vi "oa_Buffer and Compute Orbit Plot Data.vi"(5 "reset? (F)":bool, 6 "trigger pulse direction":u16(ring)=1 items=["positive going", "negative going"], 7 "tach duty":i32=1, 8 "actual samples/rev":dbl format="%.2f", 9 "revolutions":dbl format="%.2f", 10 "start":dbl format="%.2f", 11 "order waveform":dbl[][](array[numeric]) format="%.2f") -> (3 "orbit data":cluster{dbl[], dbl[]}[](array[cluster]) {"?" format="%.2f"; "?" format="%.2f"})   [LabVIEW 2017]
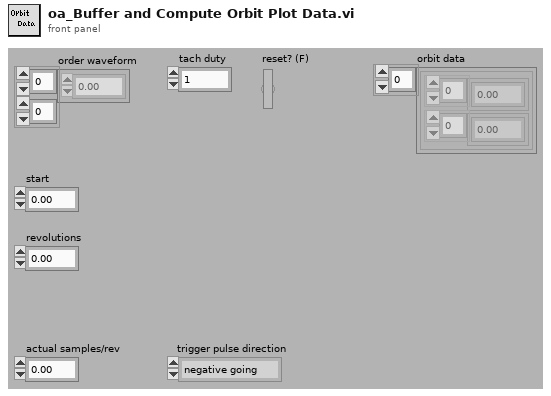
[diagram p1: front panel]
types:
  T1 = cluster{"selected order data":dbl[], "selected order data":dbl[]}
  T2 = cluster{"selected order data":dbl[], "selected order data":dbl[]}[]
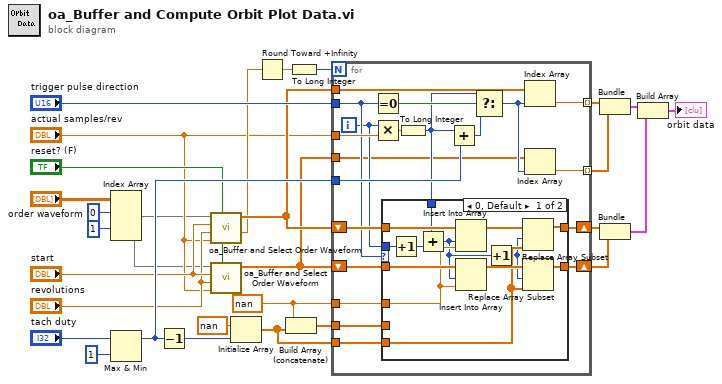
[diagram p0: block diagram]
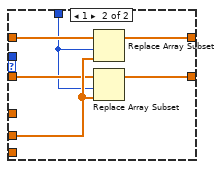
[diagram p2: hidden frame]
diagram:
  w14 = nan ("element")
  n1 = Index Array(array="order waveform", index (row) #1=0 ("index (row)"), index (row) #2=1 ("index (row)")) -> (element #1=w4:dbl[], element #2=w3:dbl[])  [unwired: 2 in]
  n2 = Max & Min(x="tach duty", y=1) -> (max(x,y)=w22:i32)  [unwired: 1 out]
  n3 = Decrement(x=w22) -> (x-1=w16:i32)
  n4 = call <vilib>:"oa_Buffer and Select Order Waveform.vi"("reset? (F)"="reset? (F)", "actual samples/rev"="actual samples/rev", "revolutions"="revolutions", "start"="start", "order data"=w4) -> ("rev out"=w11:dbl, "selected order data"=w12:dbl[])  [unwired: 5 in]
  n5 = call <vilib>:"oa_Buffer and Select Order Waveform.vi"("reset? (F)"="reset? (F)", "actual samples/rev"="actual samples/rev", "revolutions"="revolutions", "start"="start", "order data"=w3) -> ("selected order data"=w9:dbl[])  [unwired: 5 in, 1 out]
  n6 = Initialize Array(nan ("element"), w16) -> (w13:dbl[])
  n7 = Round Toward +Infinity(x=w11) -> (ceil(x): smallest int >= x=w23:dbl)
  n8 = Build Array (concatenate)(w14, w13) -> (w15:dbl[])
  n9 = To Long Integer(number=w23) -> (32bit integer=w24:i32)
  n10 = for {
    N: w24 -> [_]
    tunnel: "actual samples/rev" -> [w44]
    tunnel: "trigger pulse direction" -> [w37]
    tunnel: [w50] -> w30 mode=indexing
    tunnel: [w49] -> w29 mode=indexing
    tunnel: w22 -> [w43]
    tunnel: w15 -> [w42]
    shift-right: [w40] -> w20
    shift-left: w12 -> [w41]
    shift-right: [w39] -> w19
    shift-left: w9 -> [w31]
    tunnel: w14 -> [w36]
    tunnel: w13 -> [w34]
    tunnel: w12 -> [w33]
    tunnel: w9 -> [w32]
    i -> [w35]
    n11 = Equal To 0?(x=w37) -> (x = 0?=w48:bool)
    n12 = Multiply(x=w35, y=w44) -> (x*y=w47:dbl)
    n13 = To Long Integer(number=w47) -> (32bit integer=w38:i32)
    n14 = case shown="0, Default" w37 {
      tunnel: w42 -> [_ w69]
      tunnel: w41 -> [w63 w68]
      tunnel: [w57 w67] -> w40
      tunnel: w31 -> [w62 w66]
      tunnel: [w55 w65] -> w39
      tunnel: w38 -> [w60 w64]
      tunnel: w36 -> [w61 _]
      tunnel: w35 -> [w59 _]
      tunnel: w34 -> [w54 _]
      frame 0, Default {
        n15 = Increment(x=w59) -> (x+1=w51:i32)
        n16 = Add(x=w60, y=w51) -> (x+y=w53:i32)
        n17 = Insert Into Array(array=w63, index=w53, new element=w61) -> (w58:dbl[])
        n18 = Insert Into Array(array=w62, index=w53, new element=w61) -> (w56:dbl[])
        n19 = Increment(x=w53) -> (x+1=w52:i32)
        n20 = Replace Array Subset(array=w58, new element=w54, index=w52) -> (w57:dbl[])
        n21 = Replace Array Subset(array=w56, new element=w54, index=w52) -> (w55:dbl[])
      }
      frame 1 {
        n22 = Replace Array Subset(array=w68, new element=w69, index=w64) -> (w67:dbl[])
        n23 = Replace Array Subset(array=w66, new element=w69, index=w64) -> (w65:dbl[])
      }
    }
    n24 = Add(x=w38, y=w43) -> (x+y=w46:i32)
    n25 = Select(t=w38, s=w48, f=w46) -> (s? t:f=w45:i32)
    n26 = Index Array(array=w33, index=w45) -> (element=w50:dbl)
    n27 = Index Array(array=w32, index=w45) -> (element=w49:dbl)
  }
  n28 = Bundle(w30, w29) -> (w28:cluster{dbl[], dbl[]})  [unwired: 1 in]
  n29 = Bundle("selected order data"=w20, "selected order data"=w19) -> (w18:T1)  [unwired: 1 in]
  n30 = Build Array(w28, w18) -> (→"orbit data":T2)
